vi "Untitled 2 (SubVI).vi"(11 "position":cluster{"x":dbl, "y":dbl, "z":dbl}) -> (3 "msg out 2":string)   [LabVIEW 2016]
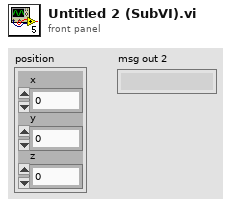
[diagram p1: front panel]
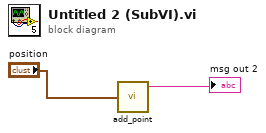
[diagram p0: block diagram]
diagram:
  n1 = call "add_point.vi"("Point"="position") -> ("msg out"=→"msg out 2":string)  [unwired: 4 in]
